vi "Meas Proc QWTB Load Algorithm.vi"(5 "qwtb unc mode ref":refnum<vi>, 6 "alg. selection changed?":bool, 7 "param table ref":refnum<vi>, 8 "error in":errorcluster, 9 "algorithm id (empty)":string, 10 "qwtb alg selector":refnum<vi>, 11 "session in":T3={"adc"={"niScope"={"channel cfg"=[], "sessions"=[], "multi cards"=FALSE, "channels"=0, "type"=enum."n/a", "memory [B/chn]"=0, "ext. clock [Hz]"=0.0, "samples count"=0, "use streaming"=FALSE, "proc setup"={"packet size [smpl]"=0, "current timeout [s]"=0.0, "blk2blk timeout [s]"=0.0, "event time"=timestamp(0 s since 1904-01-01), "temp sampl T [s]"=0.0, "data queue"=refnum, "stop notifier"=refnum, "proc ref"=refnum}, "sample width [B]"=0, "ranges [V]"=[], "trigger setup"={"coupling"=1, "level [V]"=0.0, "slope"=0, "mode"=enum."Immediate"}, "fs [Hz]"=0.0, "bitres [bit]"=0}, "3458A"={"channels"=[], "sync unit"={"VISA"="", "type"=enum."Picotest U6200A"}, "awg unit"={"type"=enum."Agilent 331xxA to 332xxA", "VISA"="", "enable 10MHz ref"=FALSE}, "sync mode"=enum."MASTER-SLAVE, MASTER clocked by TIMER", "streaming mode"=FALSE, "idn mode"=enum."Auto", "sampling mode"=enum."DCV", "Ts [s]"=0.0, "sample memory [B]"=0, "proc setup"={"channel id"=0, "packet size [smpl]"=0, "current timeout [s]"=0.0, "blk2blk timeout [s]"=0.0, "event time"=timestamp(0 s since 1904-01-01), "stop notifier"=refnum, "data queues"=[], "proc refs"=[], "bus semaphore"=refnum}, "sample size [B]"=0, "sample count"=0, "aux data"={"channel id"=0, "valid?"=[], "gain [V]"=[], "timestamp [s]"=[], "Ts [s]"=0.0, "abs timestamp"=timestamp(0 s since 1904-01-01), "t [deg C]"=[]}, "ranges [V]"=[], "aperture [s]"=0.0, "LEVEL trigger"={"edge"=enum."POS", "level [V]"=0.0, "coupling"=enum."DC"}, "trigger mode"=enum."AUTO", "measure temp.?"=FALSE, "disp mesages"=[], "shared bus?"=FALSE, "disable display?"=FALSE, "aper mode"=enum."Manual", "aper rules"=[]}, "dsdll"={"dsdll"={"dsdll path"=path "", "dsdll handle"=[], "output devices"=[], "capture devices"=[]}, "channels"=0, "device id"=0, "channel idns"=[], "proc setup"={"packet size [smpl]"=0, "current timeout [s]"=0.0, "blk2blk timeout [s]"=0.0, "event time"=timestamp(0 s since 1904-01-01), "data queue"=refnum, "stop notifier"=refnum, "proc ref"=refnum}, "samples count"=0, "fs [Hz]"=0.0}, "type"=enum."niScope", "channel idn str"=[], "aux instr idn str"=[], "modified?"=FALSE, "simadc"={"channels"=[], "range [V]"=0.0, "Ts step [s]"=0.0, "time [s]"=0.0, "fs [Hz]"=0.0, "count"=0, "smpl offset"=0, "set count"=0, "bit res"=0}, "force rst?"=FALSE, "exit mode"=enum."Immediate reset", "exit dly"=0.0, "exit tmr"=timestamp(0 s since 1904-01-01), "busy?"=FALSE, "accessed?"=FALSE, "QuADC session"={"channel cfg"=[], "sessions"=[], "multi cards"=FALSE, "channels"=0, "type"=enum."n/a", "memory [B/chn]"=0, "ext. clock [Hz]"=0.0, "samples count"=0, "use streaming"=FALSE, "proc setup"={"packet size [smpl]"=0, "current timeout [s]"=0.0, "blk2blk timeout [s]"=0.0, "event time"=timestamp(0 s since 1904-01-01), "temp sampl T [s]"=0.0, "data queue"=refnum, "stop notifier"=refnum, "proc ref"=refnum}, "sample width [B]"=0, "ranges [V]"=[], "trigger setup"={"coupling"=1, "level [V]"=0.0, "slope"=0, "mode"=enum."Immediate"}, "fs [Hz]"=0.0, "bitres [bit]"=0}}, "sequence"=[], "sequence setup"={"group setups"=[], "average cycles"=0, "range mode"=enum."Keep defaults", "fs mode"=enum."Frequency", "rng even"=0.0, "rng odd"=0.0, "folder"=path "", "name base"="", "meas id"=0, "settle [s]"=0.0}, "golpi"=refnum, "processing setup"={"mode"=enum."Raw", "call after avgs?"=FALSE, "calculate?"=FALSE, "raw mode"={"command"="", "result mode"=enum."Display console output (only Octave)", "res variable"=""}, "QWTB"={"QWTB path"=path "", "alg filter path"="", "alg ids"=[], "alg parameters"=[], "parsed parameters"=[], "selected alg id"="", "selected unc mode"=enum."None", "qwtb mcc"=100, "qwtb timeout"=90, "qwtb covg"=95.0, "qwtb ofs"=0, "qwtb lim data"=0, "multicore"={"jobs folder"=path "", "cores"=0, "max jobs"=0, "mode"=enum."Singlecore"}, "unc once?"=FALSE}}, "corrections"={"transducers"={"channels"=[], "last path"=path ""}, "digitizer"={"last path"=path "", "channel paths"=[], "channel idns"=[], "correction name"="", "channel names"=[], "folders to copy"=[], "channel valid"=[], "correction path"=path "", "correction rel path"="", "rel folders to copy"=[]}}, "assist cfg"={"P"=0, "Q"=0, "rel shift"=0.0, "ref freq"=0.0, "min fs"=0.0, "max fs tol"=0.0, "min int"=0.0, "max int"=0.0, "max err"=0.0, "max timeout"=0.0}} {"corrections"."transducers"."channels"."Phase index" min=1 step=1; "adc"."QuADC session"."trigger setup"."level [V]" format="%.2f"; "adc"."QuADC session"."trigger setup"."coupling" items=["AC"=0, "DC"=1, "HF Reject"=3, "LF Reject"=4, "AC Plus HF Reject"=1001]; "adc"."QuADC session"."channel cfg"."Clock fr. (Hz)" min=0.0 format="%#_9p"; "adc"."QuADC session"."channel cfg"."Number of JJ" min=1; "adc"."QuADC session"."channel cfg"."Range [Vpk]" min=0.0; "adc"."QuADC session"."channel cfg"."Channel" min=0; "adc"."3458A"."channels"."Range [Vpk]" min=0.0; "adc"."niScope"."trigger setup"."level [V]" format="%.2f"; "adc"."niScope"."trigger setup"."coupling" items=["AC"=0, "DC"=1, "HF Reject"=3, "LF Reject"=4, "AC Plus HF Reject"=1001]; "adc"."niScope"."channel cfg"."Range [Vpk]" min=0.0; "adc"."niScope"."channel cfg"."Channel" min=0}) -> (0 "error out":errorcluster, 1 "qwtb alg flags":T1, 2 "algorithm info":T2, 3 "session out":T3={"adc"={"niScope"={"channel cfg"=[], "sessions"=[], "multi cards"=FALSE, "channels"=0, "type"=enum."n/a", "memory [B/chn]"=0, "ext. clock [Hz]"=0.0, "samples count"=0, "use streaming"=FALSE, "proc setup"={"packet size [smpl]"=0, "current timeout [s]"=0.0, "blk2blk timeout [s]"=0.0, "event time"=timestamp(0 s since 1904-01-01), "temp sampl T [s]"=0.0, "data queue"=refnum, "stop notifier"=refnum, "proc ref"=refnum}, "sample width [B]"=0, "ranges [V]"=[], "trigger setup"={"coupling"=1, "level [V]"=0.0, "slope"=0, "mode"=enum."Immediate"}, "fs [Hz]"=0.0, "bitres [bit]"=0}, "3458A"={"channels"=[], "sync unit"={"VISA"="", "type"=enum."Picotest U6200A"}, "awg unit"={"type"=enum."Agilent 331xxA to 332xxA", "VISA"="", "enable 10MHz ref"=FALSE}, "sync mode"=enum."MASTER-SLAVE, MASTER clocked by TIMER", "streaming mode"=FALSE, "idn mode"=enum."Auto", "sampling mode"=enum."DCV", "Ts [s]"=0.0, "sample memory [B]"=0, "proc setup"={"channel id"=0, "packet size [smpl]"=0, "current timeout [s]"=0.0, "blk2blk timeout [s]"=0.0, "event time"=timestamp(0 s since 1904-01-01), "stop notifier"=refnum, "data queues"=[], "proc refs"=[], "bus semaphore"=refnum}, "sample size [B]"=0, "sample count"=0, "aux data"={"channel id"=0, "valid?"=[], "gain [V]"=[], "timestamp [s]"=[], "Ts [s]"=0.0, "abs timestamp"=timestamp(0 s since 1904-01-01), "t [deg C]"=[]}, "ranges [V]"=[], "aperture [s]"=0.0, "LEVEL trigger"={"edge"=enum."POS", "level [V]"=0.0, "coupling"=enum."DC"}, "trigger mode"=enum."AUTO", "measure temp.?"=FALSE, "disp mesages"=[], "shared bus?"=FALSE, "disable display?"=FALSE, "aper mode"=enum."Manual", "aper rules"=[]}, "dsdll"={"dsdll"={"dsdll path"=path "", "dsdll handle"=[], "output devices"=[], "capture devices"=[]}, "channels"=0, "device id"=0, "channel idns"=[], "proc setup"={"packet size [smpl]"=0, "current timeout [s]"=0.0, "blk2blk timeout [s]"=0.0, "event time"=timestamp(0 s since 1904-01-01), "data queue"=refnum, "stop notifier"=refnum, "proc ref"=refnum}, "samples count"=0, "fs [Hz]"=0.0}, "type"=enum."niScope", "channel idn str"=[], "aux instr idn str"=[], "modified?"=FALSE, "simadc"={"channels"=[], "range [V]"=0.0, "Ts step [s]"=0.0, "time [s]"=0.0, "fs [Hz]"=0.0, "count"=0, "smpl offset"=0, "set count"=0, "bit res"=0}, "force rst?"=FALSE, "exit mode"=enum."Immediate reset", "exit dly"=0.0, "exit tmr"=timestamp(0 s since 1904-01-01), "busy?"=FALSE, "accessed?"=FALSE, "QuADC session"={"channel cfg"=[], "sessions"=[], "multi cards"=FALSE, "channels"=0, "type"=enum."n/a", "memory [B/chn]"=0, "ext. clock [Hz]"=0.0, "samples count"=0, "use streaming"=FALSE, "proc setup"={"packet size [smpl]"=0, "current timeout [s]"=0.0, "blk2blk timeout [s]"=0.0, "event time"=timestamp(0 s since 1904-01-01), "temp sampl T [s]"=0.0, "data queue"=refnum, "stop notifier"=refnum, "proc ref"=refnum}, "sample width [B]"=0, "ranges [V]"=[], "trigger setup"={"coupling"=1, "level [V]"=0.0, "slope"=0, "mode"=enum."Immediate"}, "fs [Hz]"=0.0, "bitres [bit]"=0}}, "sequence"=[], "sequence setup"={"group setups"=[], "average cycles"=0, "range mode"=enum."Keep defaults", "fs mode"=enum."Frequency", "rng even"=0.0, "rng odd"=0.0, "folder"=path "", "name base"="", "meas id"=0, "settle [s]"=0.0}, "golpi"=refnum, "processing setup"={"mode"=enum."Raw", "call after avgs?"=FALSE, "calculate?"=FALSE, "raw mode"={"command"="", "result mode"=enum."Display console output (only Octave)", "res variable"=""}, "QWTB"={"QWTB path"=path "", "alg filter path"="", "alg ids"=[], "alg parameters"=[], "parsed parameters"=[], "selected alg id"="", "selected unc mode"=enum."None", "qwtb mcc"=100, "qwtb timeout"=90, "qwtb covg"=95.0, "qwtb ofs"=0, "qwtb lim data"=0, "multicore"={"jobs folder"=path "", "cores"=0, "max jobs"=0, "mode"=enum."Singlecore"}, "unc once?"=FALSE}}, "corrections"={"transducers"={"channels"=[], "last path"=path ""}, "digitizer"={"last path"=path "", "channel paths"=[], "channel idns"=[], "correction name"="", "channel names"=[], "folders to copy"=[], "channel valid"=[], "correction path"=path "", "correction rel path"="", "rel folders to copy"=[]}}, "assist cfg"={"P"=0, "Q"=0, "rel shift"=0.0, "ref freq"=0.0, "min fs"=0.0, "max fs tol"=0.0, "min int"=0.0, "max int"=0.0, "max err"=0.0, "max timeout"=0.0}} {"corrections"."transducers"."channels"."Phase index" min=1 step=1; "adc"."QuADC session"."trigger setup"."level [V]" format="%.2f"; "adc"."QuADC session"."trigger setup"."coupling" items=["AC"=0, "DC"=1, "HF Reject"=3, "LF Reject"=4, "AC Plus HF Reject"=1001]; "adc"."QuADC session"."channel cfg"."Clock fr. (Hz)" min=0.0 format="%#_9p"; "adc"."QuADC session"."channel cfg"."Number of JJ" min=1; "adc"."QuADC session"."channel cfg"."Range [Vpk]" min=0.0; "adc"."QuADC session"."channel cfg"."Channel" min=0; "adc"."3458A"."channels"."Range [Vpk]" min=0.0; "adc"."niScope"."trigger setup"."level [V]" format="%.2f"; "adc"."niScope"."trigger setup"."coupling" items=["AC"=0, "DC"=1, "HF Reject"=3, "LF Reject"=4, "AC Plus HF Reject"=1001]; "adc"."niScope"."channel cfg"."Range [Vpk]" min=0.0; "adc"."niScope"."channel cfg"."Channel" min=0}, 4 "parameters table":string)   [LabVIEW 2018]
doc: "This VI will load information for selected QWTB algorithm. The algorithm index is index of previously loaded algorithm list starting from 1. Index 0 is invalid selection/no selection."
uses:
  Meas Session.ctl
  adc/ADC Session.ctl
  drivers/niScope/niScope Session.ctl
  drivers/niScope/niScope Virtual Channel Config.ctl
  drivers/niScope/niScope Virtual Channel Mode.ctl
  drivers/niScope/niScope Virtual Channel Input Z.ctl
  drivers/niScope/niScope Virtual Channel Coupling.ctl
  drivers/niScope/niScope Type.ctl
  drivers/niScope/niScope Digitizing Process Options.ctl
  drivers/niScope/niScope Data Packet.ctl
  drivers/niScope/niScope Trigger Setup.ctl
  <instrlib>/niScope/Controls/niScope trigger coupling.ctl
  <instrlib>/niScope/Controls/niScope trigger slope.ctl
  drivers/DMM/3458A Digitizer Session.ctl
  drivers/DMM/3458A Virtual Channel Config.ctl
  drivers/Counter/Counter Session.ctl
  drivers/Counter/Counter Type.ctl
  drivers/AWG/AWG Session.ctl
  drivers/AWG/AWG Type.ctl
  drivers/DMM/3458A Sync Mode.ctl
  drivers/DMM/3458A Idn Mode.ctl
  drivers/DMM/3458A Digitizing Low Levels/Configure/Sampling Mode.ctl
  drivers/DMM/3458A Digitizing Process Options.ctl
  drivers/DMM/3458A Data Packet.ctl
  drivers/DMM/3458A Aux Record Data.ctl
  drivers/DMM/3458A Digitizing Low Levels/Configure/Level Setup.ctl
  drivers/DMM/3458A Digitizing Low Levels/Configure/First Sample Trigger.ctl
  drivers/DMM/3458A Aperture Selection Mode.ctl
  drivers/dsdll/DSDLL Session.ctl
  drivers/dsdll/dsdll source distribution/dsdll_instance.ctl
  drivers/dsdll/dsdll source distribution/dsdll_device_record.ctl
  drivers/dsdll/DSDLL Process Config.ctl
  drivers/dsdll/DSDLL Data Packet.ctl
  adc/ADC Type.ctl
  drivers/simulated_adc/SimAdc Config.ctl
  drivers/simulated_adc/SimAdc Channel Cfg.ctl
  adc/ADC On Close Action.ctl
  drivers/Quatsch_driver/QuADCDriver/QuADC Session.ctl
  drivers/Quatsch_driver/QuADCDriver/QuADC Virtual Channel Config.ctl
  drivers/Quatsch_driver/QuADCDriver/QuADC Virtual Channel Mode.ctl
  drivers/Quatsch_driver/QuADCDriver/QuADC Virtual Channel Input Z.ctl
  drivers/Quatsch_driver/QuADCDriver/QuADC Virtual Channel Coupling.ctl
  drivers/Quatsch_driver/QuADCDriver/QuADC Type.ctl
  drivers/Quatsch_driver/QuADCDriver/QuADC Digitizing Process Options.ctl
  drivers/Quatsch_driver/QuADCDriver/QuADC Data Packet.ctl
  drivers/Quatsch_driver/QuADCDriver/QuADC Trigger Setup.ctl
  Meas Sequence Item.ctl
  Meas Sampling Configuration.ctl
  adc/ADC Trig Config.ctl
  adc/ADC Trig Mode Source.ctl
  adc/ADC Trig Coupling.ctl
  adc/ADC Trig Slope.ctl
  Meas Proc QWTB Algorithm Parameter Data.ctl
  Meas Sequence Configuration.ctl
  Meas Range Mode.ctl
  Meas Sampling Rate Mode.ctl
  octave/golpi/mpc/golpi_session_ref.ctl
  octave/golpi/mpc/golpi_session.ctl
  octave/golpi/GOLPI Library.lvlibp/Public/GOLPI reference Type Def.ctl
  octave/golpi/GOLPI Library.lvlibp/LV Process source distribution/Pipe Handle.ctl
  Meas Process Config.ctl
  Meas Process Mode.ctl
  Meas Process Raw Config.ctl
  Meas Process Raw Result Mode.ctl
  Meas Proc QWTB Setup.ctl
  Meas Proc QWTB Uncertainty Mode.ctl
  Meas Proc QWTB Multicore Setup.ctl
  Meas Proc QWTB Multicore Type.ctl
  Corrections/Corr Setup.ctl
  Corrections/Corr Tranducer Item.ctl
  Corrections/Corr Digitizers.ctl
  Assist/Assist Panel Setup.ctl
  Meas Proc QWTB Algorithm Info.ctl
  Meas Proc QWTB Algorithm Flags.ctl
  octave/golpi/GOLPI Library.lvlibp/Private/Get Variable - polymorph parts/Get String.vi
  octave/golpi/GOLPI Library.lvlibp/Private/Get Variable - polymorph parts/Get 1D Array Double.vi
  octave/golpi/mpc/GOLPI Multi Process.lvlib
  octave/golpi/GOLPI Library.lvlibp
  drivers/niScope/niScope Virtual Digitizer.lvlib
  drivers/DMM/3458A Virtual Digitizer.lvlib
  drivers/Counter/Counter.lvlib
  drivers/AWG/AWG.lvlib
  drivers/DMM/3458A Digitizing Low Levels/3458A Digitizing Low Levels.lvlib
  drivers/dsdll/DSDLL Virtual Digitizer.lvlib
  octave/golpi/GOLPI Library.lvlibp/LV Process source distribution/LV Process library.lvlib
  drivers/Quatsch_driver/QuADCDriver/QuADC Virtual Digitizer.lvlib
  drivers/dsdll/dsdll source distribution/dsdll.lvlib
panel:
  # "ADC:"
  # "IP Address"
  # "."
  # "."
  # "."
  # ":"
  # "ADC:"
  # "IP Address"
  # "."
  # "."
  # "."
  # ":"
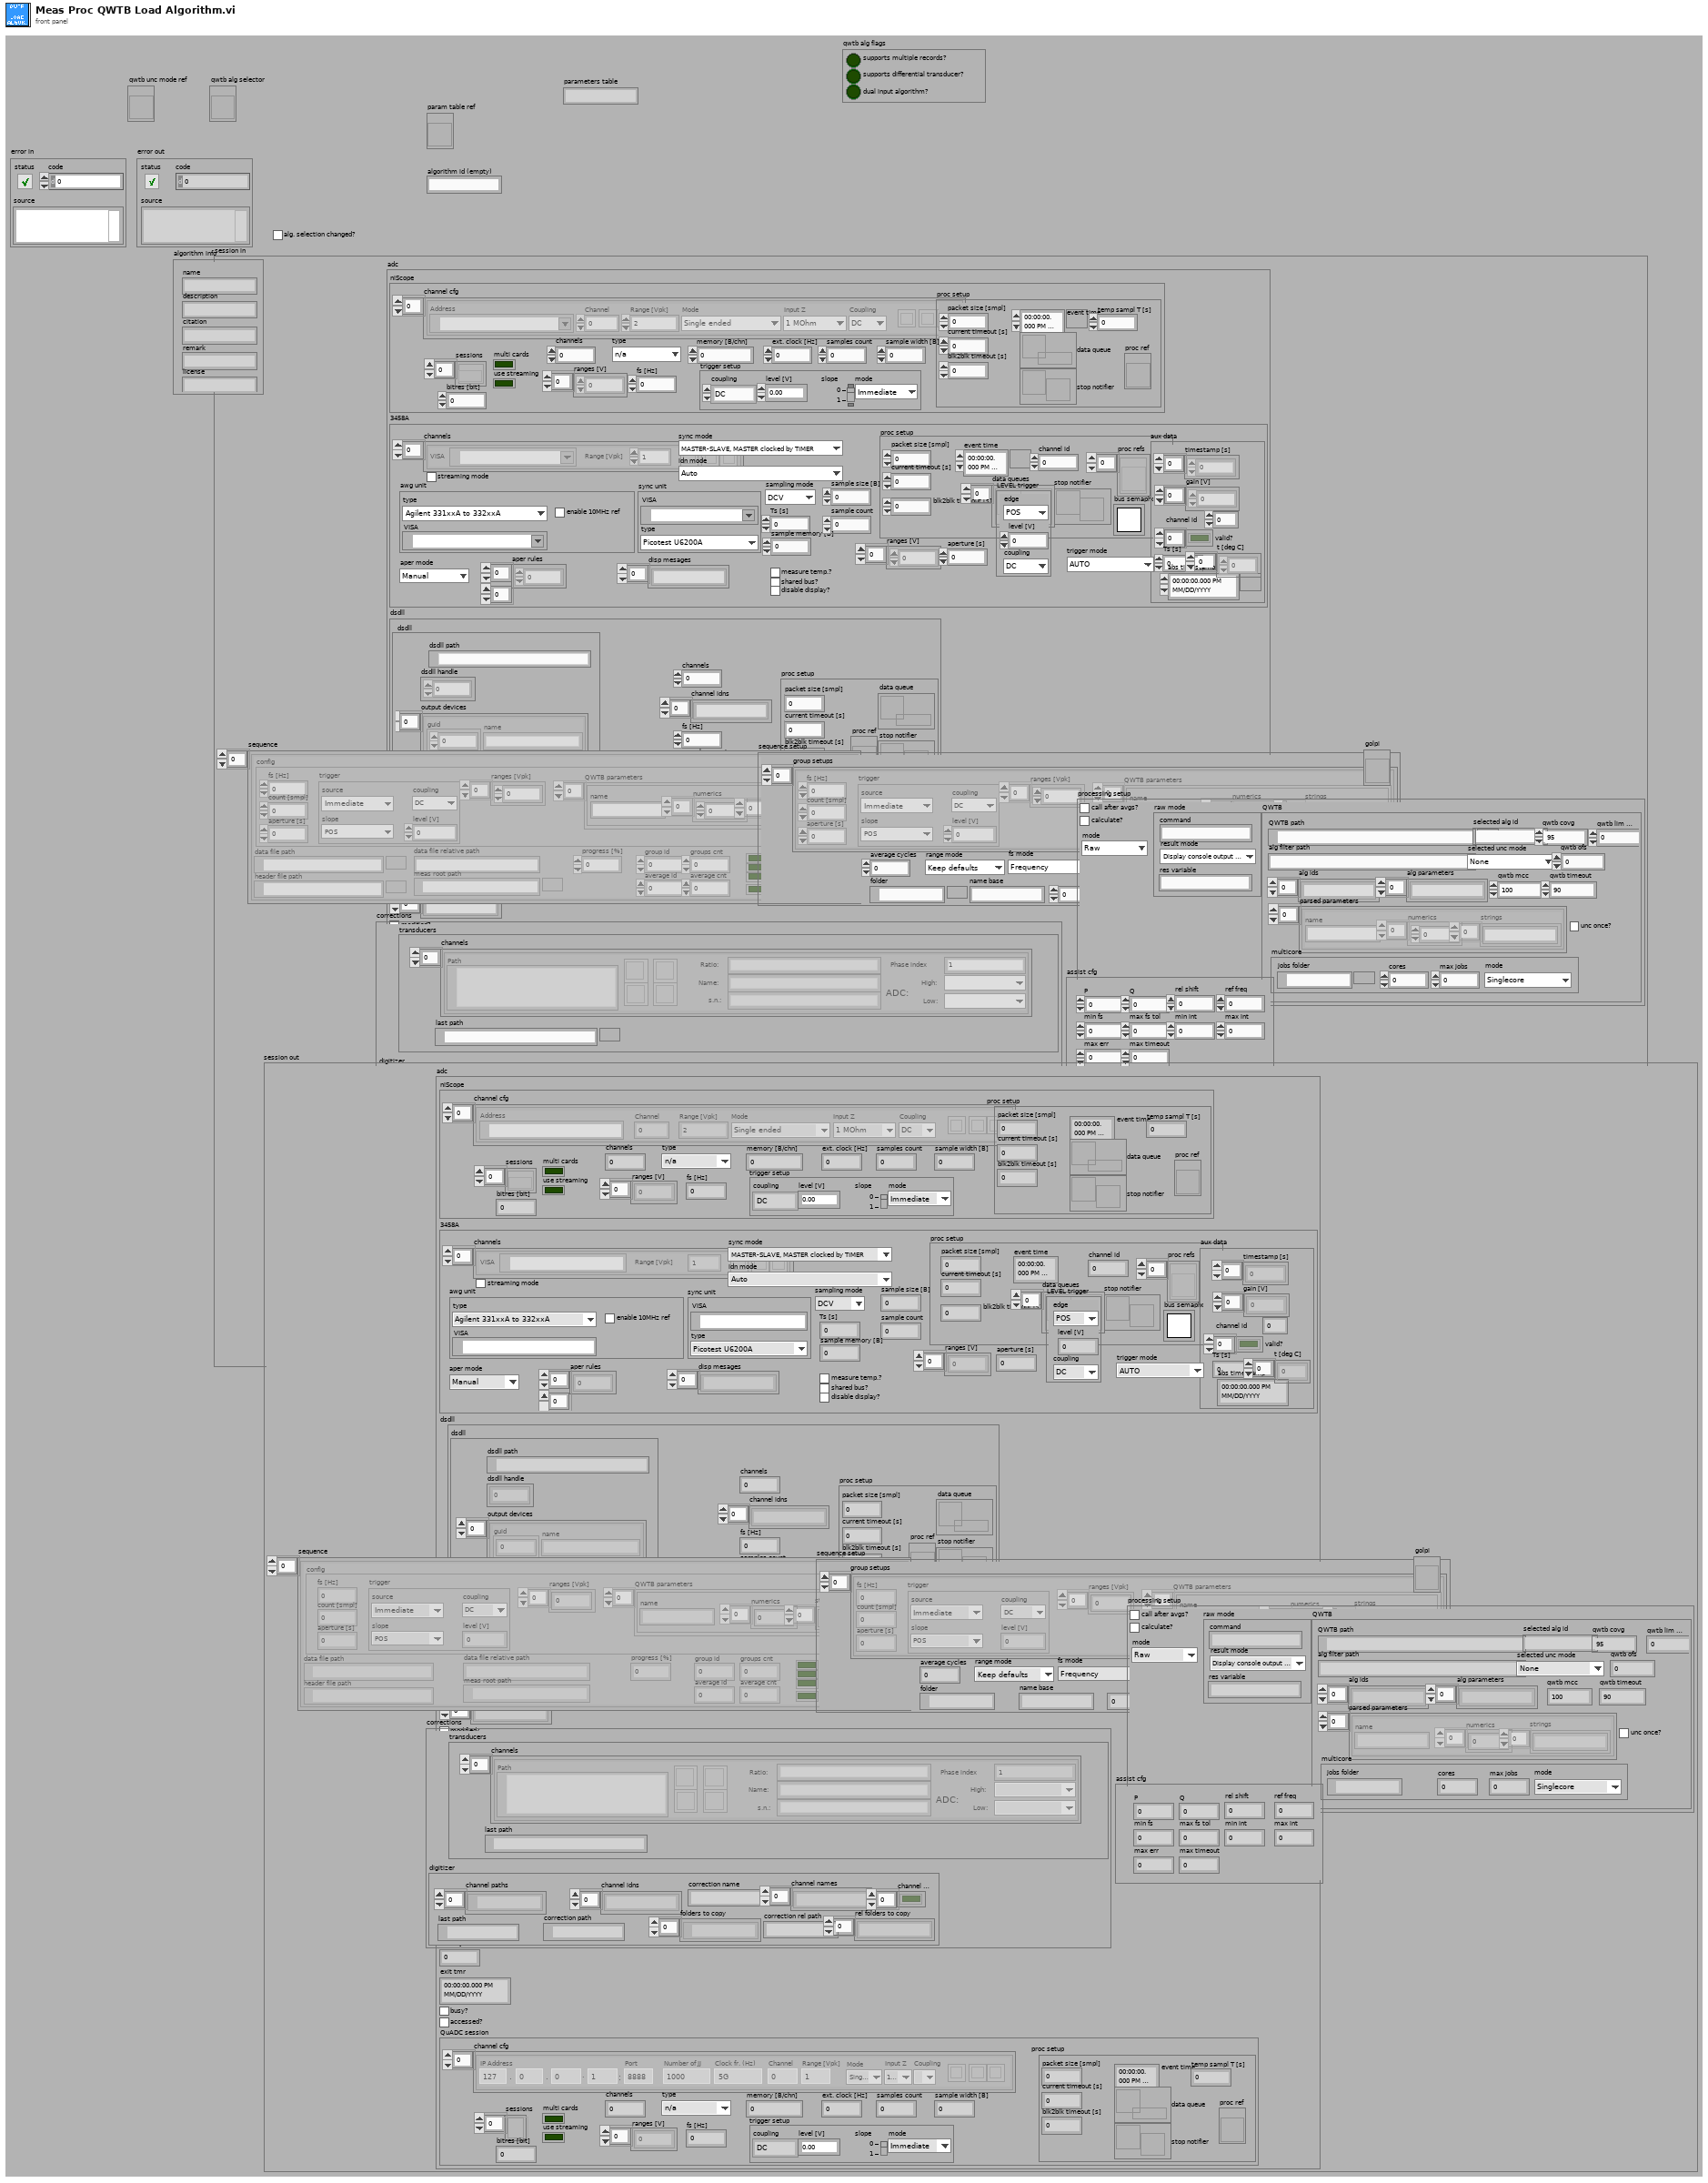
[diagram p1: front panel]
types:
  T1 = typedef "Meas Proc QWTB Algorithm Flags.ctl" = cluster{"supports multiple records?":bool, "supports differential transducer?":bool, "dual input algorithm?":bool}
  T2 = typedef "Meas Proc QWTB Algorithm Info.ctl" = cluster{"name":string, "description":string, "citation":string, "remark":string, "license":string}
  T3 = typedef "Meas Session.ctl" = cluster{"adc":T4, "sequence":T46[], "sequence setup":T53, "golpi":T56, "processing setup":T57, "corrections":T65, "assist cfg":T68}
  T4 = typedef "ADC Session.ctl" = cluster{"niScope":T5, "3458A":T15, "dsdll":T30, "type":T34, "channel idn str":string[], "aux instr idn str":string[], "modified?":bool, "simadc":T35, "force rst?":bool, "exit mode":T37, "exit dly":dbl, "exit tmr":timestamp, "busy?":bool, "accessed?":bool, "QuADC session":T38}
  T5 = typedef "niScope Virtual Digitizer.lvlib/niScope Session.ctl" = cluster{"channel cfg":T6[], "sessions":refnum<k20>[], "multi cards":bool, "channels":i32, "type":T10, "memory [B/chn]":i32, "ext. clock [Hz]":dbl, "samples count":i64, "use streaming":bool, "proc setup":T11, "sample width [B]":i32, "ranges [V]":dbl[], "trigger setup":T12, "fs [Hz]":dbl, "bitres [bit]":i32}
  T6 = typedef "niScope Virtual Digitizer.lvlib/niScope Virtual Channel Config.ctl" = cluster{"Address":refnum<k15>, "Channel":i32, "Mode":T7, "Input Z":T8, "Coupling":T9, "Range [Vpk]":dbl, "btn clr":bool, "btn up":bool, "btn down":bool}
  T7 = typedef "niScope Virtual Digitizer.lvlib/niScope Virtual Channel Mode.ctl" = enum16{"Single ended", "Unbal. differential", "Differential"}
  T8 = typedef "niScope Virtual Digitizer.lvlib/niScope Virtual Channel Input Z.ctl" = enum16{"1 MOhm", "50 Ohm"}
  T9 = typedef "niScope Virtual Digitizer.lvlib/niScope Virtual Channel Coupling.ctl" = enum16{"AC", "DC", "GND"}
  T10 = typedef "niScope Virtual Digitizer.lvlib/niScope Type.ctl" = enum16{"n/a", "5922"}
  T11 = typedef "niScope Virtual Digitizer.lvlib/niScope Digitizing Process Options.ctl" = cluster{"packet size [smpl]":i64, "current timeout [s]":dbl, "blk2blk timeout [s]":dbl, "event time":timestamp, "temp sampl T [s]":dbl, "data queue":refnum<queue>, "stop notifier":refnum<notifier>, "proc ref":refnum<vi>}
  T12 = typedef "niScope Virtual Digitizer.lvlib/niScope Trigger Setup.ctl" = cluster{"coupling":T13, "level [V]":dbl, "slope":T14, "mode":enum16{"Immediate", "External", "Level"}}
  T13 = typedef "niScope trigger coupling.ctl" = u16
  T14 = typedef "niScope trigger slope.ctl" = i32
  T15 = typedef "3458A Virtual Digitizer.lvlib/3458A Digitizer Session.ctl" = cluster{"channels":T16[], "sync unit":T17, "awg unit":T19, "sync mode":T21, "streaming mode":bool, "idn mode":T22, "sampling mode":T23, "Ts [s]":dbl, "sample memory [B]":i32, "proc setup":T24, "sample size [B]":i32, "sample count":i32, "aux data":T26, "ranges [V]":dbl[], "aperture [s]":dbl, "LEVEL trigger":T27, "trigger mode":T28, "measure temp.?":bool, "disp mesages":string[], "shared bus?":bool, "disable display?":bool, "aper mode":T29, "aper rules":dbl[][]}
  T16 = typedef "3458A Virtual Digitizer.lvlib/3458A Virtual Channel Config.ctl" = cluster{"VISA":refnum<visa-resource-name>, "Range [Vpk]":dbl, "btn clr":bool, "btn up":bool, "btn down":bool}
  T17 = typedef "Counter.lvlib/Counter Session.ctl" = cluster{"VISA":refnum<visa-resource-name>, "type":T18}
  T18 = typedef "Counter.lvlib/Counter Type.ctl" = enum16{"Picotest U6200A", "dummy"}
  T19 = typedef "AWG.lvlib/AWG Session.ctl" = cluster{"type":T20, "VISA":refnum<visa-resource-name>, "enable 10MHz ref":bool}
  T20 = typedef "AWG.lvlib/AWG Type.ctl" = enum16{"Agilent 331xxA to 332xxA", "Agilent 335xxA to 336xxA", "Tektronix AFG3101C", "dummy"}
  T21 = typedef "3458A Virtual Digitizer.lvlib/3458A Sync Mode.ctl" = enum16{"MASTER-SLAVE, MASTER clocked by TIMER", "MASTER-SLAVE, MASTER clocked by AWG", "ALL clocked by AWG", "MASTER-SLAVE, ALL clocked by TIMER", "ALL clocked by AWG with DFLL"}
  T22 = typedef "3458A Virtual Digitizer.lvlib/3458A Idn Mode.ctl" = enum16{"Auto", "Sequential (chn A, chn B, ...)", "From calibration string"}
  T23 = typedef "3458A Virtual Digitizer.lvlib/3458A Digitizing Low Levels.lvlib/Sampling Mode.ctl" = enum16{"DCV", "DSDC", "DSAC"}
  T24 = typedef "3458A Virtual Digitizer.lvlib/3458A Digitizing Process Options.ctl" = cluster{"channel id":i32, "packet size [smpl]":i32, "current timeout [s]":dbl, "blk2blk timeout [s]":dbl, "event time":timestamp, "stop notifier":refnum<notifier>, "data queues":refnum<queue>[], "proc refs":refnum<vi>[], "bus semaphore":T25}
  T25 = typedef "Semaphore RefNum" = refnum<k1>
  T26 = typedef "3458A Virtual Digitizer.lvlib/3458A Aux Record Data.ctl" = cluster{"channel id":i32, "valid?":bool[], "gain [V]":dbl[], "timestamp [s]":dbl[], "Ts [s]":dbl, "abs timestamp":timestamp, "t [deg C]":dbl[]}
  T27 = typedef "3458A Virtual Digitizer.lvlib/3458A Digitizing Low Levels.lvlib/Level Setup.ctl" = cluster{"edge":enum16{"POS", "NEG"}, "level [V]":dbl, "coupling":enum16{"DC", "AC"}}
  T28 = typedef "3458A Virtual Digitizer.lvlib/3458A Digitizing Low Levels.lvlib/First Sample Trigger.ctl" = enum16{"AUTO", "EXT", "SYN", "SGL", "HOLD", "LEVEL"}
  T29 = typedef "3458A Virtual Digitizer.lvlib/3458A Aperture Selection Mode.ctl" = enum16{"Manual", "Maximum", "Table"}
  T30 = typedef "DSDLL Virtual Digitizer.lvlib/DSDLL Session.ctl" = cluster{"dsdll":T31, "channels":i32, "device id":i32, "channel idns":string[], "proc setup":T33, "samples count":i32, "fs [Hz]":dbl}
  T31 = typedef "dsdll.lvlib/dsdll_instance.ctl" = cluster{"dsdll path":path, "dsdll handle":u8[], "output devices":T32[], "capture devices":T32[]}
  T32 = typedef "dsdll.lvlib/dsdll_device_record.ctl" = cluster{"guid":u8[], "name":string}
  T33 = typedef "DSDLL Virtual Digitizer.lvlib/DSDLL Process Config.ctl" = cluster{"packet size [smpl]":i32, "current timeout [s]":dbl, "blk2blk timeout [s]":dbl, "event time":timestamp, "data queue":refnum<queue>, "stop notifier":refnum<notifier>, "proc ref":refnum<vi>}
  T34 = typedef "ADC Type.ctl" = enum16{"niScope", "3458A", "DirectSound DLL", "dummy", "QuADC"}
  T35 = typedef "SimAdc Config.ctl" = cluster{"channels":T36[], "range [V]":dbl, "Ts step [s]":dbl, "time [s]":dbl, "fs [Hz]":dbl, "count":i64, "smpl offset":i64, "set count":i64, "bit res":i32}
  T36 = typedef "SimAdc Channel Cfg.ctl" = cluster{"harmonics":dbl[][], "btn clear":bool, "noise":dbl, "fundamental [Hz]":dbl}
  T37 = typedef "ADC On Close Action.ctl" = enum16{"Immediate reset", "Delayed reset"}
  T38 = typedef "QuADC Virtual Digitizer.lvlib/QuADC Session.ctl" = cluster{"channel cfg":T39[], "sessions":refnum<k5>[], "multi cards":bool, "channels":i32, "type":T43, "memory [B/chn]":i32, "ext. clock [Hz]":dbl, "samples count":i64, "use streaming":bool, "proc setup":T44, "sample width [B]":i32, "ranges [V]":dbl[], "trigger setup":T45, "fs [Hz]":dbl, "bitres [bit]":i32}
  T39 = typedef "QuADC Virtual Digitizer.lvlib/QuADC Virtual Channel Config.ctl" = cluster{"Channel":i32, "Mode":T40, "Input Z":T41, "Coupling":T42, "Range [Vpk]":dbl, "btn clr":bool, "btn up":bool, "btn down":bool, "IP address A":u8, "IP address B":u8, "IP address C":u8, "IP address D":u8, "Port":u16, "Number of JJ":u32, "Clock fr. (Hz)":dbl}
  T40 = typedef "QuADC Virtual Digitizer.lvlib/QuADC Virtual Channel Mode.ctl" = enum16{"Single ended", "Unbal. differential", "Differential"}
  T41 = typedef "QuADC Virtual Digitizer.lvlib/QuADC Virtual Channel Input Z.ctl" = enum16{"1 MOhm", "50 Ohm"}
  T42 = typedef "QuADC Virtual Digitizer.lvlib/QuADC Virtual Channel Coupling.ctl" = enum16{"AC", "DC", "GND"}
  T43 = typedef "QuADC Virtual Digitizer.lvlib/QuADC Type.ctl" = enum16{"n/a", "v1"}
  T44 = typedef "QuADC Virtual Digitizer.lvlib/QuADC Digitizing Process Options.ctl" = cluster{"packet size [smpl]":i64, "current timeout [s]":dbl, "blk2blk timeout [s]":dbl, "event time":timestamp, "temp sampl T [s]":dbl, "data queue":refnum<queue>, "stop notifier":refnum<notifier>, "proc ref":refnum<vi>}
  T45 = typedef "QuADC Virtual Digitizer.lvlib/QuADC Trigger Setup.ctl" = cluster{"coupling":T13, "level [V]":dbl, "slope":T14, "mode":enum16{"Immediate", "External", "Level"}}
  T46 = typedef "Meas Sequence Item.ctl" = cluster{"config":T47, "data file path":path, "header file path":path, "group id":i32, "average id":i32, "group done?":bool, "adc modified?":bool, "source modified?":bool, "progress [%]":dbl, "groups cnt":i32, "average cnt":i32, "data file relative path":string, "meas root path":path, "calculate?":bool}
  T47 = typedef "Meas Sampling Configuration.ctl" = cluster{"fs [Hz]":dbl, "count [smpl]":i64, "aperture [s]":dbl, "trigger":T48, "ranges [Vpk]":dbl[], "QWTB parameters":T52[]}
  T48 = typedef "ADC Trig Config.ctl" = cluster{"source":T49, "level [V]":dbl, "coupling":T50, "slope":T51}
  T49 = typedef "ADC Trig Mode Source.ctl" = enum16{"Immediate", "External", "Level"}
  T50 = typedef "ADC Trig Coupling.ctl" = enum16{"DC", "AC"}
  T51 = typedef "ADC Trig Slope.ctl" = enum16{"POS", "NEG"}
  T52 = typedef "Meas Proc QWTB Algorithm Parameter Data.ctl" = cluster{"name":string, "numerics":dbl[], "strings":string[]}
  T53 = typedef "Meas Sequence Configuration.ctl" = cluster{"group setups":T47[], "average cycles":i32, "range mode":T54, "fs mode":T55, "rng even":dbl, "rng odd":dbl, "folder":path, "name base":string, "meas id":i32, "settle [s]":dbl}
  T54 = typedef "Meas Range Mode.ctl" = enum16{"Keep defaults", "Set All channels", "Set Odd and Even channels"}
  T55 = typedef "Meas Sampling Rate Mode.ctl" = enum16{"Frequency", "Period"}
  T56 = typedef "GOLPI Multi Process.lvlib/golpi_session_ref.ctl" = refnum<vi>
  T57 = typedef "Meas Process Config.ctl" = cluster{"mode":T58, "call after avgs?":bool, "calculate?":bool, "raw mode":T59, "QWTB":T61}
  T58 = typedef "Meas Process Mode.ctl" = enum16{"Raw", "QWTB"}
  T59 = typedef "Meas Process Raw Config.ctl" = cluster{"command":string, "result mode":T60, "res variable":string}
  T60 = typedef "Meas Process Raw Result Mode.ctl" = enum16{"Display console output (only Octave)", "Display string variable", "Display result file %respath%"}
  T61 = typedef "Meas Proc QWTB Setup.ctl" = cluster{"QWTB path":path, "alg filter path":string, "alg ids":string[], "alg parameters":string[], "parsed parameters":T52[], "selected alg id":string, "selected unc mode":T62, "qwtb mcc":i32, "qwtb timeout":i32, "qwtb covg":dbl, "qwtb ofs":i64, "qwtb lim data":i64, "multicore":T63, "unc once?":bool}
  T62 = typedef "Meas Proc QWTB Uncertainty Mode.ctl" = enum16{"None", "GUF", "Monte Carlo"}
  T63 = typedef "Meas Proc QWTB Multicore Setup.ctl" = cluster{"jobs folder":path, "cores":i32, "max jobs":i32, "mode":T64}
  T64 = typedef "Meas Proc QWTB Multicore Type.ctl" = enum16{"Singlecore", "Multicore", "Multistation"}
  T65 = typedef "Corr Setup.ctl" = cluster{"transducers":cluster{"channels":T66[], "last path":path}, "digitizer":T67}
  T66 = typedef "Corr Tranducer Item.ctl" = cluster{"Path":path, "Ratio:":string, "Name:":string, "btn rem":bool, "btn up":bool, "btn down":bool, "s.n.:":string, "btn open":bool, "ratio o/i":dbl, "chn hi":u16, "chn lo":u16, "Phase index":i32}
  T67 = typedef "Corr Digitizers.ctl" = cluster{"last path":path, "channel paths":path[], "channel idns":string[], "correction name":string, "channel names":string[], "folders to copy":path[], "channel valid":bool[], "correction path":path, "correction rel path":string, "rel folders to copy":string[]}
  T68 = typedef "Assist Panel Setup.ctl" = cluster{"P":i32, "Q":i32, "rel shift":dbl, "ref freq":dbl, "min fs":dbl, "max fs tol":dbl, "min int":dbl, "max int":dbl, "max err":dbl, "max timeout":dbl}
  T69 = typedef "GOLPI Library.lvlibp/GOLPI reference Type Def.ctl" = cluster{"pipe handle":T70, "fast read timeout [ms]":u32, "fast read settle time [ms]":u32, "fast read to multiple [ms]":u32, "max elements per input line":u32, "slow read timeout [ms]":u32, "stdin double format specifier":string, "max elements per stdout output column":u32, "console mode bitstream":bool, "bitstream first read timeout [ms]":u32, "bitstream read timeout [ms]":u32, "struct transfer possible":bool, "matlab mode":bool}
  T70 = typedef "GOLPI Library.lvlibp/LV Process library.lvlib/Pipe Handle.ctl" = cluster{"lv_proc.dll file path":path, "process instance handle":u32[], "debug mode":bool, "debug data":cluster{"time":timestamp, "stdin":bool, "data":string}[]}
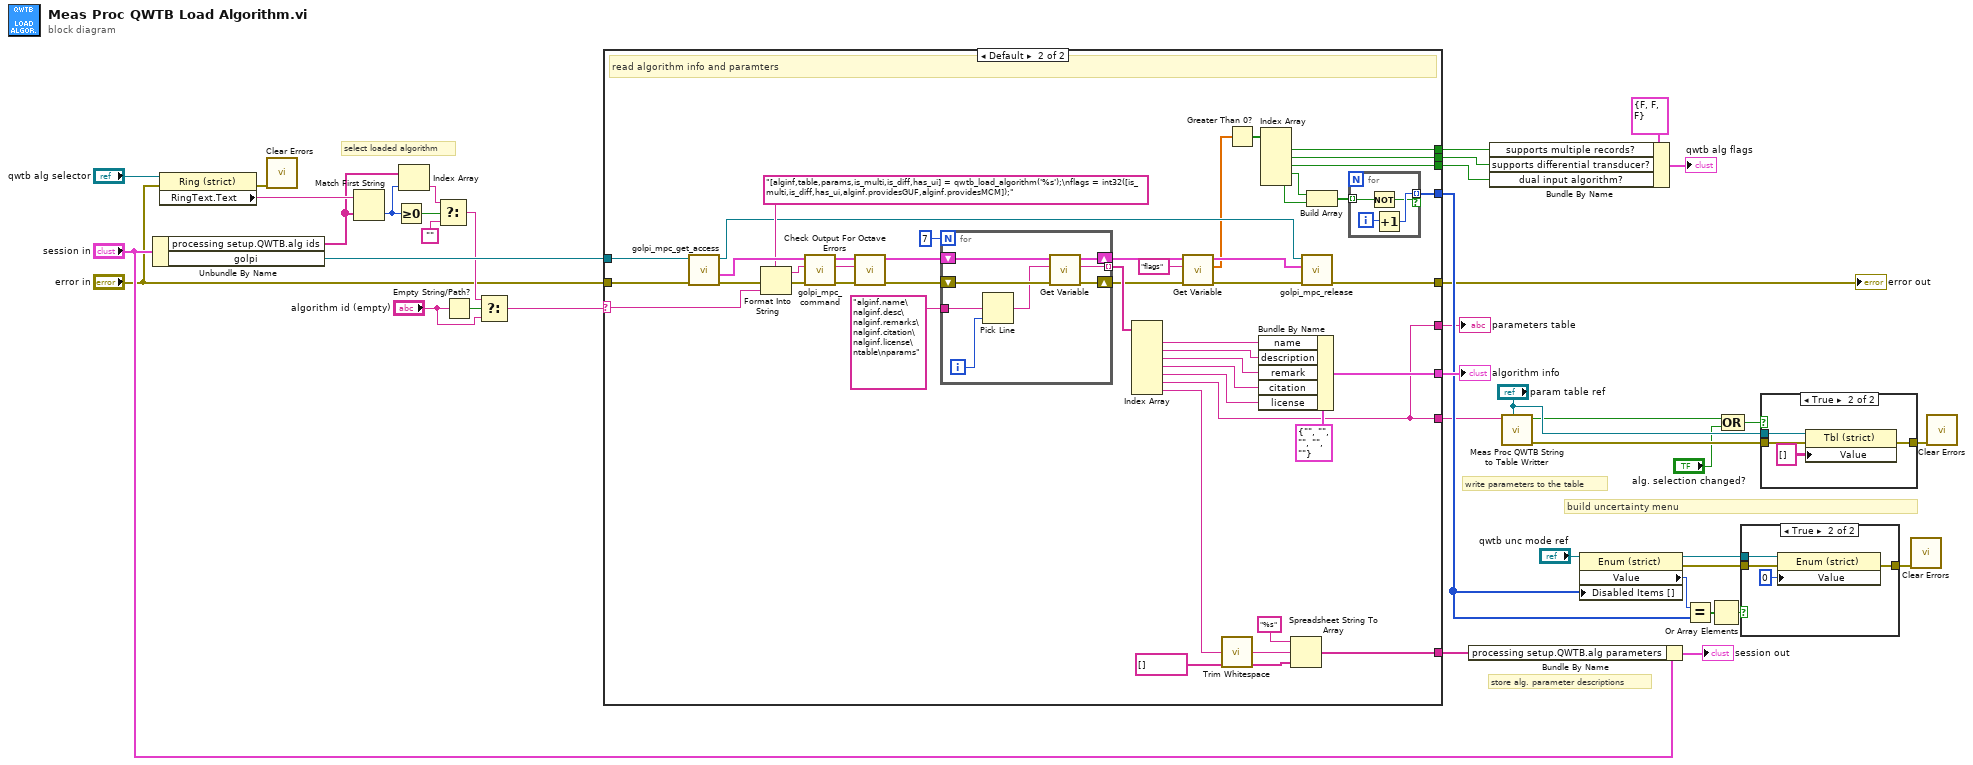
[diagram p0: block diagram]
diagram:
  # "select loaded algorithm"
  # "store alg. parameter descriptions"
  # "build uncertainty menu"
  # "write parameters to the table"
  n1 = Unbundle By Name("session in") -> ("processing setup.QWTB.alg ids"=w12:string[], "golpi"=w40:T56)
  n2 = property class="Ring (strict)"(reference="qwtb alg selector", error in="error in") -> (error out=w4:errorcluster, "RingText.Text"=w15:string)  [unwired: 1 out]
  n3 = call <vilib>:"Clear Errors.vi"("error in (no error)"=w4) -> ()  [unwired: 5 in, 2 out]
  n4 = Match First String(2:w12, 3:w15) -> (0:w11:i32)  [unwired: 1 out]
  n5 = Greater Or Equal To 0?(x=w11) -> (x >= 0?=w14:bool)
  n6 = Index Array(array=w12, index=w11) -> (element=w13:string)
  n7 = Select(t=w13, s=w14, f="") -> (s? t:f=w8:string)
  n8 = Empty String/Path?(string/path="algorithm id (empty)") -> (empty?=w9:bool)
  n9 = Select(t=w8, s=w9, f="algorithm id (empty)") -> (s? t:f=w6:string)
  n10 = case shown="Default" w6 {
    selector: w6 -> [_ w43]
    tunnel: "error in" -> [w41 w85]
    tunnel: w40 -> [_ w83]
    tunnel: [w41 w78] -> w2
    tunnel: [_ w68] -> w39
    tunnel: [_ w42] -> w21
    tunnel: [_ w63] -> w32
    tunnel: [_ w51] -> w29
    tunnel: [_ w50] -> w28
    tunnel: [_ w49] -> w27
    tunnel: [_ w44] -> w24
    tunnel: [_ w42] -> w1
    frame "" {
    }
    frame Default {
      # "read algorithm info and paramters"
      n11 = call "golpi_mpc_get_access.vi"("error in"=w85, "golpi session ref"=w83) -> ("error out"=w81:errorcluster, "GOLPI ref out"=w84:T69, "golpi session ref out (copy)"=w79:T56)  [unwired: 4 in, 3 out]
      n12 = Format Into String(format string="[alginf,table,params,is_multi,is_diff,has_ui] = qwtb_load_algorithm('%s');\nflags = int32([is_multi,is_diff,has_ui,alginf.providesGUF,alginf.providesMCM]);" ("command"), error in=w81, w43) -> (resulting string=w77:string, error out=w82:errorcluster)  [unwired: 1 in]
      n13 = call "golpi_mpc_command.vi"("error in"=w82, "command"=w77, "GOLPI ref in"=w84) -> ("error out"=w62:errorcluster, "read buffer"=w61:string, "GOLPI ref. out"=w59:T69)  [unwired: 6 in]
      n14 = call "Check Output For Octave Errors.vi"("error in"=w62, "read buffer"=w61) -> ("error out"=w60:errorcluster)  [unwired: 9 in]
      n15 = for {
        N: 7 -> [_]
        tunnel: "alginf.name\nalginf.desc\nalginf.remarks\nalginf.citation\nalginf.license\ntable\nparams" ("variable name") -> [w94]
        tunnel: [w92] -> w75 mode=indexing
        shift-right: [w90] -> w57
        shift-left: w59 -> [w96]
        shift-right: [w91] -> w58
        shift-left: w60 -> [w97]
        i -> [w93]
        n16 = Pick Line(multi-line string=w94, line index=w93) -> (output string=w95:string)  [unwired: 1 in]
        n17 = call-poly "Get Variable.vi"("error in"=w97, "variable name"=w95, "GOLPI ref. in"=w96) -> ("error out"=w91:errorcluster, "value"=w92:string, "GOLPI ref. out"=w90:T69)  [unwired: 6 in]
      }
      n18 = Index Array(array=w75) -> (element #1=w73:string, element #2=w72:string, element #3=w71:string, element #4=w70:string, element #5=w69:string, element #6=w42:string, element #7=w48:string)  [unwired: 7 in]
      n19 = call-poly "Get Variable.vi"("error in"=w58, "variable name"="flags", "GOLPI ref. in"=w57) -> ("error out"=w56:errorcluster, "value"=w53:dbl[], "GOLPI ref. out"=w55:T69)  [unwired: 6 in]
      n20 = call <vilib>:"Trim Whitespace.vi"("string"=w48) -> ("trimmed string"=w66:string)  [unwired: 1 in]
      n21 = Greater Than 0?(x=w53) -> (x > 0?=w52:bool[])
      n22 = Bundle By Name(cluster=T2 {"name"="", "description"="", "citation"="", "remark"="", "license"=""} ("alg info"), "name"=w73, "description"=w72, "remark"=w71, "citation"=w70, "license"=w69) -> (w68:T2)
      n23 = Index Array(array=w52) -> (element #1=w51:bool, element #2=w50:bool, element #3=w49:bool, element #4=w47:bool, element #5=w46:bool)  [unwired: 5 in]
      n24 = Spreadsheet String To Array(format string="%s", spreadsheet string=w66, array type (2D Dbl)=string[] []) -> (array=w63:string[])  [unwired: 1 in]
      n25 = call "golpi_mpc_release.vi"("error in"=w56, "golpi ref or golpi session in"=w55, "golpi session ref"=w79) -> ("error out"=w78:errorcluster)  [unwired: 7 in, 1 out]
      n26 = Build Array(w47, w46) -> (w45:bool[])
      n27 = for {
        tunnel: w45 -> [w87] mode=indexing
        tunnel: [w88] -> w44 mode=indexing if=w86
        i -> [w89]
        n28 = Not(x=w87) -> (.not. x?=w86:bool)
        n29 = Increment(x=w89) -> (x+1=w88:i32)
      }
    }
  }
  "error out" <- w2
  "algorithm info" <- w39
  "parameters table" <- w1
  n30 = Bundle By Name(cluster="session in", "processing setup.QWTB.alg parameters"=w32) -> (→"session out":T3)
  n31 = Bundle By Name(cluster=T1 {"supports multiple records?"=FALSE, "supports differential transducer?"=FALSE, "dual input algorithm?"=FALSE} ("qwtb alg flags"), "supports multiple records?"=w29, "supports differential transducer?"=w28, "dual input algorithm?"=w27) -> (→"qwtb alg flags":T1)
  n32 = call "Meas Proc QWTB String to Table Writter.vi"("param table ref"="param table ref", "content csv string"=w21) -> ("error out"=w22:errorcluster, "row header changed?"=w17:bool)  [unwired: 8 in]
  n33 = property class="Enum (strict)"(reference="qwtb unc mode ref", "Disabled Items []"=w24) -> (reference out=w36:refnum<vi>, error out=w37:errorcluster, "Value"=w38:T62)  [unwired: 1 in]
  n34 = Equal?(x=w38, y=w24) -> (x = y?=w35:bool[])
  n35 = Or Array Elements(Boolean array=w35) -> (logical OR=w23:bool)
  n36 = Compound Arithmetic op=OR(w17, "alg. selection changed?") -> (w19:bool)
  n37 = case shown="True" w23 {
    tunnel: w37 -> [w98 w102]
    tunnel: w36 -> [_ w101]
    tunnel: [w98 w99] -> w34
    frame False {
    }
    frame True {
      n38 = property class="Enum (strict)"(reference=w101, error in=w102, "Value"=u16 0) -> (error out=w99:errorcluster)  [unwired: 1 out]
    }
  }
  n39 = case shown="True" w19 {
    tunnel: w22 -> [w103 w107]
    tunnel: "param table ref" -> [_ w106]
    tunnel: [w103 w104] -> w3
    frame False {
    }
    frame True {
      n40 = property class="Tbl (strict)"(reference=w106, error in=w107, "Value"=string[][] []) -> (error out=w104:errorcluster)  [unwired: 1 out]
    }
  }
  n41 = call <vilib>:"Clear Errors.vi"("error in (no error)"=w34) -> ()  [unwired: 5 in, 2 out]
  n42 = call <vilib>:"Clear Errors.vi"("error in (no error)"=w3) -> ()  [unwired: 5 in, 2 out]
